vi "DeviceBan.vi"(7 "Available":bool, 8 "error in":errorcluster caption="错误输入（无错误）", 9 "CAN通路":T2(ring)=enum."CAN3", 10 "ViewCtl":T1, 11 "设备":T3) -> (0 "error out":errorcluster caption="错误输出")   [LabVIEW 2013]
uses:
  Ctl/DeviceCtl.ctl
  Ctl/ViewCtl.ctl
  USBCAN/DevType.ctl
panel:
  # "ms"
  # "ms"
  # "s"
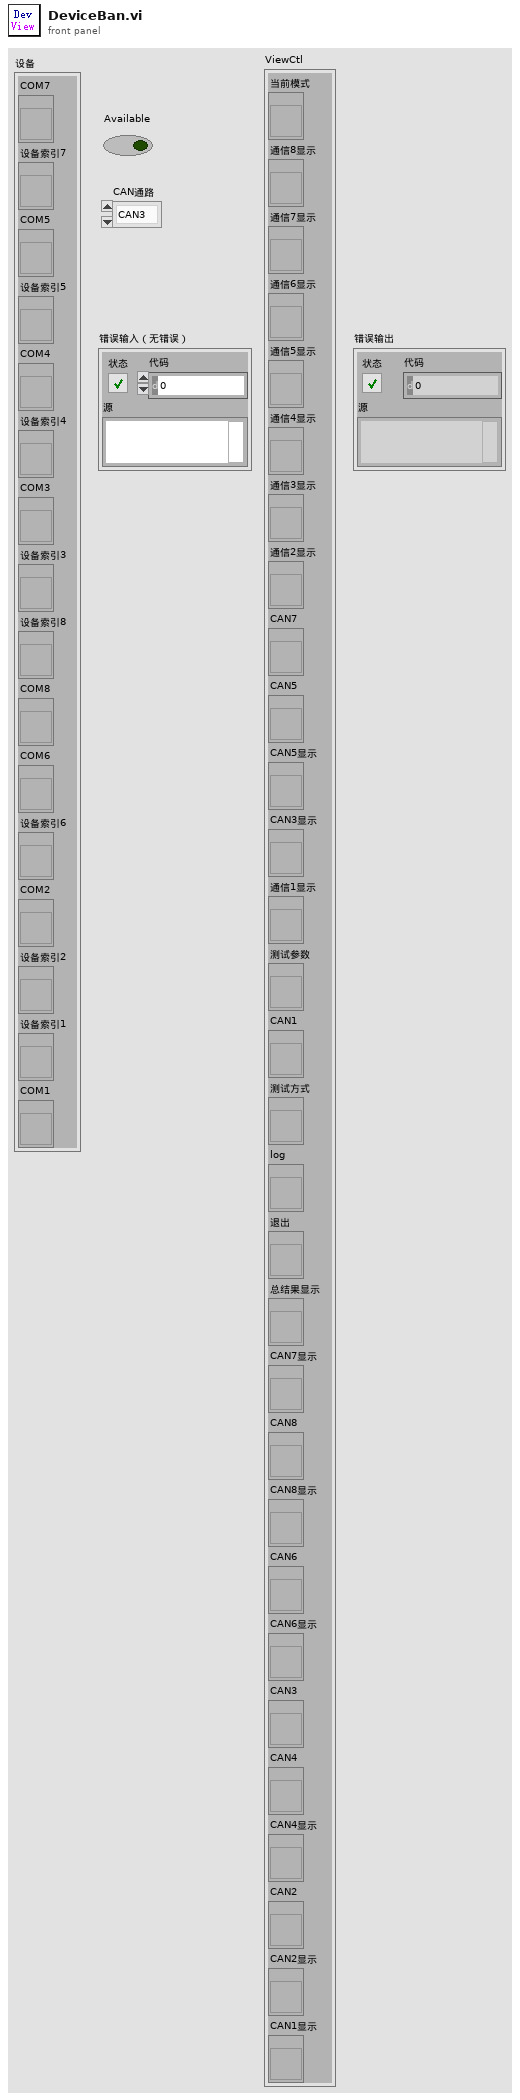
[diagram p1: front panel]
types:
  T1 = typedef "ViewCtl.ctl" = cluster{"当前模式":refnum<vi>, "通信8显示":refnum<vi>, "通信7显示":refnum<vi>, "通信6显示":refnum<vi>, "通信5显示":refnum<vi>, "通信4显示":refnum<vi>, "通信3显示":refnum<vi>, "通信2显示":refnum<vi>, "CAN7":refnum<vi>, "CAN5":refnum<vi>, "CAN5显示":refnum<vi>, "CAN3显示":refnum<vi>, "通信1显示":refnum<vi>, "测试参数":refnum<vi>, "CAN1":refnum<vi>, "测试方式":refnum<vi>, "log":refnum<vi>, "退出":refnum<vi>, "总结果显示":refnum<vi>, "CAN7显示":refnum<vi>, "CAN8":refnum<vi>, "CAN8显示":refnum<vi>, "CAN6":refnum<vi>, "CAN6显示":refnum<vi>, "CAN3":refnum<vi>, "CAN4":refnum<vi>, "CAN4显示":refnum<vi>, "CAN2":refnum<vi>, "CAN2显示":refnum<vi>, "CAN1显示":refnum<vi>}
  T2 = enum16{"CAN1", "CAN2", "CAN3", "CAN4", "CAN5", "CAN6", "CAN7", "CAN8"}
  T3 = typedef "DeviceCtl.ctl" = cluster{"COM7":refnum<vi>, "设备索引7":refnum<vi>, "COM5":refnum<vi>, "设备索引5":refnum<vi>, "COM4":refnum<vi>, "设备索引4":refnum<vi>, "COM3":refnum<vi>, "设备索引3":refnum<vi>, "设备索引8":refnum<vi>, "COM8":refnum<vi>, "COM6":refnum<vi>, "设备索引6":refnum<vi>, "COM2":refnum<vi>, "设备索引2":refnum<vi>, "设备索引1":refnum<vi>, "COM1":refnum<vi>}
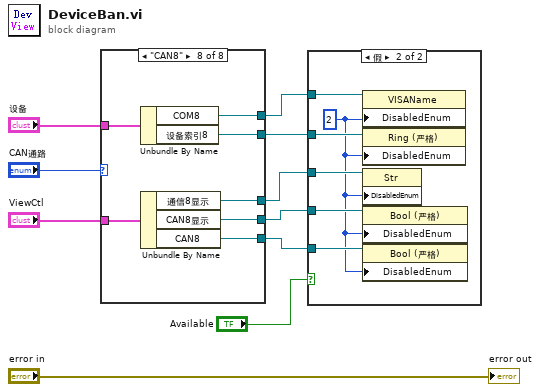
[diagram p0: block diagram]
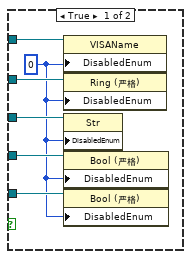
[diagram p2: hidden frame]
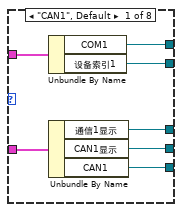
[diagram p3: hidden frame]
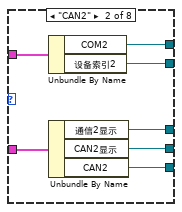
[diagram p4: hidden frame]
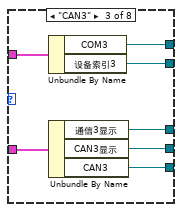
[diagram p5: hidden frame]
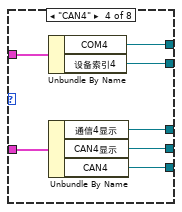
[diagram p6: hidden frame]
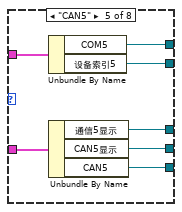
[diagram p7: hidden frame]
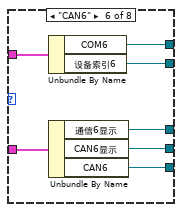
[diagram p8: hidden frame]
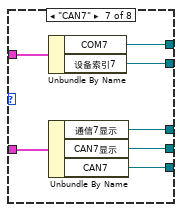
[diagram p9: hidden frame]
diagram:
  n1 = case shown="\"CAN8\"" "CAN通路" {
    tunnel: "设备" -> [w17 w24 w31 w38 w45 w52 w59 w66]
    tunnel: "ViewCtl" -> [w16 w23 w30 w37 w44 w51 w58 w65]
    tunnel: [w15 w22 w29 w36 w43 w50 w57 w64] -> w7
    tunnel: [w14 w21 w28 w35 w42 w49 w56 w63] -> w6
    tunnel: [w13 w20 w27 w34 w41 w48 w55 w62] -> w5
    tunnel: [w12 w19 w26 w33 w40 w47 w54 w61] -> w4
    tunnel: [w11 w18 w25 w32 w39 w46 w53 w60] -> w3
    frame "CAN1", Default {
      n2 = Unbundle By Name(w17) -> ("COM1"=w15:refnum<vi>, "设备索引1"=w14:refnum<vi>)
      n3 = Unbundle By Name(w16) -> ("通信1显示"=w13:refnum<vi>, "CAN1显示"=w12:refnum<vi>, "CAN1"=w11:refnum<vi>)
    }
    frame "CAN2" {
      n4 = Unbundle By Name(w24) -> ("COM2"=w22:refnum<vi>, "设备索引2"=w21:refnum<vi>)
      n5 = Unbundle By Name(w23) -> ("通信2显示"=w20:refnum<vi>, "CAN2显示"=w19:refnum<vi>, "CAN2"=w18:refnum<vi>)
    }
    frame "CAN3" {
      n6 = Unbundle By Name(w31) -> ("COM3"=w29:refnum<vi>, "设备索引3"=w28:refnum<vi>)
      n7 = Unbundle By Name(w30) -> ("通信3显示"=w27:refnum<vi>, "CAN3显示"=w26:refnum<vi>, "CAN3"=w25:refnum<vi>)
    }
    frame "CAN4" {
      n8 = Unbundle By Name(w38) -> ("COM4"=w36:refnum<vi>, "设备索引4"=w35:refnum<vi>)
      n9 = Unbundle By Name(w37) -> ("通信4显示"=w34:refnum<vi>, "CAN4显示"=w33:refnum<vi>, "CAN4"=w32:refnum<vi>)
    }
    frame "CAN5" {
      n10 = Unbundle By Name(w45) -> ("COM5"=w43:refnum<vi>, "设备索引5"=w42:refnum<vi>)
      n11 = Unbundle By Name(w44) -> ("通信5显示"=w41:refnum<vi>, "CAN5显示"=w40:refnum<vi>, "CAN5"=w39:refnum<vi>)
    }
    frame "CAN6" {
      n12 = Unbundle By Name(w52) -> ("COM6"=w50:refnum<vi>, "设备索引6"=w49:refnum<vi>)
      n13 = Unbundle By Name(w51) -> ("通信6显示"=w48:refnum<vi>, "CAN6显示"=w47:refnum<vi>, "CAN6"=w46:refnum<vi>)
    }
    frame "CAN7" {
      n14 = Unbundle By Name(w59) -> ("COM7"=w57:refnum<vi>, "设备索引7"=w56:refnum<vi>)
      n15 = Unbundle By Name(w58) -> ("通信7显示"=w55:refnum<vi>, "CAN7显示"=w54:refnum<vi>, "CAN7"=w53:refnum<vi>)
    }
    frame "CAN8" {
      n16 = Unbundle By Name(w66) -> ("COM8"=w64:refnum<vi>, "设备索引8"=w63:refnum<vi>)
      n17 = Unbundle By Name(w65) -> ("通信8显示"=w62:refnum<vi>, "CAN8显示"=w61:refnum<vi>, "CAN8"=w60:refnum<vi>)
    }
  }
  n18 = case shown="假" "Available" {
    tunnel: w7 -> [w72 w78]
    tunnel: w6 -> [w71 w77]
    tunnel: w5 -> [w70 w76]
    tunnel: w4 -> [w69 w75]
    tunnel: w3 -> [w68 w74]
    frame True {
      w67 = 0
      n19 = property class="VISAName"(reference=w72, "DisabledEnum"=w67) -> ()  [unwired: 1 in, 2 out]
      n20 = property class="Ring (严格)"(reference=w71, "DisabledEnum"=w67) -> ()  [unwired: 1 in, 2 out]
      n21 = property class="Str"(reference=w70, "DisabledEnum"=w67) -> ()  [unwired: 1 in, 2 out]
      n22 = property class="Bool (严格)"(reference=w69, "DisabledEnum"=w67) -> ()  [unwired: 1 in, 2 out]
      n23 = property class="Bool (严格)"(reference=w68, "DisabledEnum"=w67) -> ()  [unwired: 1 in, 2 out]
    }
    frame False {
      w73 = 2
      n24 = property class="VISAName"(reference=w78, "DisabledEnum"=w73) -> ()  [unwired: 1 in, 2 out]
      n25 = property class="Ring (严格)"(reference=w77, "DisabledEnum"=w73) -> ()  [unwired: 1 in, 2 out]
      n26 = property class="Str"(reference=w76, "DisabledEnum"=w73) -> ()  [unwired: 1 in, 2 out]
      n27 = property class="Bool (严格)"(reference=w75, "DisabledEnum"=w73) -> ()  [unwired: 1 in, 2 out]
      n28 = property class="Bool (严格)"(reference=w74, "DisabledEnum"=w73) -> ()  [unwired: 1 in, 2 out]
    }
  }
  "error out" <- "error in"
